vi "Get Data.vi"(8 "error in":errorcluster, 11 "TSI 3022 in":refnum<class "TSI 3022.lvclass">) -> (0 "error out":errorcluster, 2 "Data Out":refnum<class "CPC Data.lvclass">, 3 "TSI 3022 out":refnum<class "TSI 3022.lvclass">)   [LabVIEW 2014, in "TSI 3022.lvclass"]
uses:
  TSI 3022.lvclass
  TSI 3025/TSI 3025.lvclass
  Data/CPC Data.lvclass
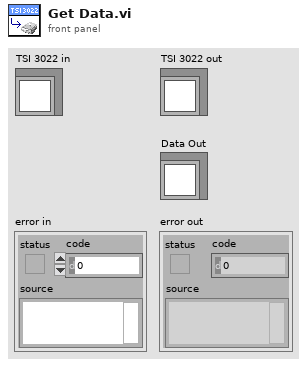
[diagram p1: front panel]
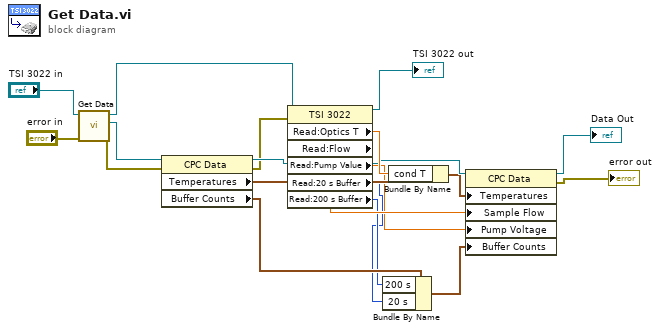
[diagram p0: block diagram]
diagram:
  n1 = call-parent "Get Data.vi"("error in"="error in", "TSI 3025 in"="TSI 3022 in") -> ("error out"=w3:errorcluster, "Data Out"=w17:refnum<class "CPC Data.lvclass">, "TSI 3025 out"=w16:refnum<class "TSI 3022.lvclass">)  [unwired: 7 in]
  n2 = property class="CPC Data"(reference=w17, error in=w3) -> (reference out=w12:refnum<class "CPC Data.lvclass">, error out=w4:errorcluster, "Temperatures"=w15:cluster{"cond T":dbl, "sat T":dbl, "opt T":dbl}, "Buffer Counts"=w8:cluster{"200 s":u32, "20 s":u32, "1 s":u32})
  n3 = property class="TSI 3022"(reference=w16, error in=w4) -> (reference out=→"TSI 3022 out":refnum<class "TSI 3022.lvclass">, "Read:Optics T"=w14:dbl, "Read:Flow"=w10:dbl, "Read:Pump Value"=w9:dbl, "Read:20 s Buffer"=w6:i32, "Read:200 s Buffer"=w7:i32)  [unwired: 1 out]
  n4 = Bundle By Name(cluster=w8, "200 s"=w7, "20 s"=w6) -> (w5:cluster{"200 s":u32, "20 s":u32, "1 s":u32})
  n5 = Bundle By Name(cluster=w15, "cond T"=w14) -> (w11:cluster{"cond T":dbl, "sat T":dbl, "opt T":dbl})
  n6 = property class="CPC Data"(reference=w12, "Temperatures"=w11, "Sample Flow"=w10, "Pump Voltage"=w9, "Buffer Counts"=w5) -> (reference out=→"Data Out":refnum<class "CPC Data.lvclass">, error out=→"error out":errorcluster)  [unwired: 1 in]
